vi "COMTRADE Open.vi"(5 "include information file? (F)":bool, 7 "include header file? (F)":bool, 8 "error in (no error)":errorcluster, 10 "open mode":T1(ring), 11 "configuration file path":path) -> (0 "error out":errorcluster, 3 "task out":T2 {"public inf content"."Event Information"."min sample number" max=9999999999; "public inf content"."Event Information"."max sample number" max=9999999999; "config info"."nrates" max=999; "config info"."status channel info"."Dn" min=1 max=999999; "config info"."analog channel info"."An" min=1 max=999999; "config info"."trigger timestamp" format="%<%H:%M:%S%6u\n%d/%m/%Y>T"; "config info"."initial timestamp" format="%<%H:%M:%S%6u\n%d/%m/%Y>T"; "config info"."##D" max=999999; "config info"."##A" max=999999; "config info"."TT" min=1 max=999999; "config info"."rev_year" min=1999.0 max=1999.0})   [LabVIEW 2013, in "NI_EP_COMTRADE.lvlib"]
doc: "Opens a .cfg and the corresponding .dat file for reading or writing. You also can use this VI to create a new file or replace an existing file. Set <B>include header file?</B> or <B>include information file?</B> to TRUE if you also want to create or open a .hdr or .inf file. Use the COMTRADE Close VI to close references to the files. IEEE Std C37.111-1999 specifies that a filename must not exceed eight characters. However, this VI accepts filenames that have more than eight characters, but returns a warning message."
uses:
  <vilib>/addons/Electrical Power/File IO/NI_EP_COMTRADE.lvlib
  <vilib>/addons/Electrical Power/File IO/COMTRADE/typedefs/ep_Task.ctl
  <vilib>/addons/Electrical Power/File IO/COMTRADE/typedefs/ep_Config Info.ctl
  <vilib>/addons/Electrical Power/File IO/COMTRADE/typedefs/ep_Analog Channel Info.ctl
  <vilib>/addons/Electrical Power/File IO/COMTRADE/typedefs/ep_Status Channel Info.ctl
  <vilib>/addons/Electrical Power/File IO/COMTRADE/typedefs/ep_File Format.ctl
  <vilib>/addons/Electrical Power/File IO/COMTRADE/typedefs/ep_Public Inf Content.ctl
  <vilib>/addons/Electrical Power/File IO/COMTRADE/typedefs/ep_Public Event Inf.ctl
  <vilib>/addons/Electrical Power/File IO/COMTRADE/typedefs/ep_Private Inf Content.ctl
  <vilib>/Platform/storage/lvStorage.llb/_openFunction.ctl
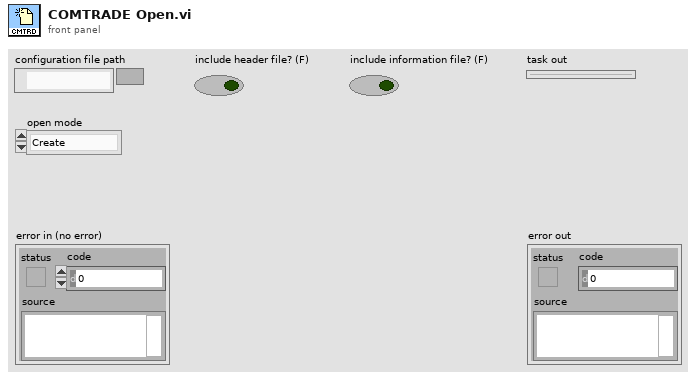
[diagram p1: front panel]
types:
  T1 = enum16{"Create", "Create or replace", "Open (read only)"}
  T2 = typedef "NI_EP_COMTRADE.lvlib/ep_Task.ctl" = cluster{"file refnums":refnum<file>[], "Data Object":refnum<k20>, "config info":T3, "public inf content":T7, "private inf content":T9, "internal buffers":cluster{"start index":u32, "config to public inf":enum16{"disabled", "enabled", "buffered"}, "static config info":string, "static file_des record inf":string, "static file_des channel inf":string, "public inf":string, "private inf":string}}
  T3 = typedef "NI_EP_COMTRADE.lvlib/ep_Config Info.ctl" = cluster{"station_name":string, "rec_dev_id":string, "rev_year":dbl, "TT":u32, "##A":u32, "##D":u32, "analog channel info":T4[], "status channel info":T5[], "lf":sgl, "nrates":u16, "samp info":cluster{"samp":sgl, "endsamp":u32}[], "initial timestamp":timestamp, "trigger timestamp":timestamp, "ft":T6, "timemult":sgl}
  T4 = typedef "NI_EP_COMTRADE.lvlib/ep_Analog Channel Info.ctl" = cluster{"An":u32, "ch_id":string, "ph":string, "ccbm":string, "uu":string, "a":sgl, "b":sgl, "skew":sgl, "min":i32, "max":i32, "primary":sgl, "secondary":sgl, "PS":enum16{"P", "S"}}
  T5 = typedef "NI_EP_COMTRADE.lvlib/ep_Status Channel Info.ctl" = cluster{"Dn":u32, "ch_id":string, "ph":string, "ccbm":string, "Y":bool}
  T6 = typedef "NI_EP_COMTRADE.lvlib/ep_File Format.ctl" = enum16{"ASCII", "Binary"}
  T7 = typedef "NI_EP_COMTRADE.lvlib/ep_Public Inf Content.ctl" = cluster{"Source":string, "Record Type":enum16{"Fault", "Unknown", "Misoperation", "Close", "Trip", "Reclose", "Power swing", "Simulation"}, "Phase ID":string, "Event Description":string, "Device ID":string, "Distance of Fault":dbl, "Distance Unit":enum16{"Miles", "Kilometers", "Percent of line", "Percent of setting", "Ohms"}, "Max_Current":dbl, "Min_Current":dbl, "Max_Voltage":dbl, "Min_Voltage":dbl, "EventNoteCount":u32, "Event Information":T8[]}
  T8 = typedef "NI_EP_COMTRADE.lvlib/ep_Public Event Inf.ctl" = cluster{"channel number":u32, "max value":dbl, "min value":dbl, "max sample number":u64, "min sample number":u64, "max sample text":string[], "min sample text":string[]}
  T9 = typedef "NI_EP_COMTRADE.lvlib/ep_Private Inf Content.ctl" = cluster{"Section Header":string, "Entry Names":string[], "Entry Values":string[]}[]
  T10 = enum16{"open", "replace", "create", "open or create", "replace or create", "replace or create with confirmation"}
  T11 = typedef "_openFunction.ctl" = enum16{"open", "open or create", "create or replace", "create", "open (read only)"}
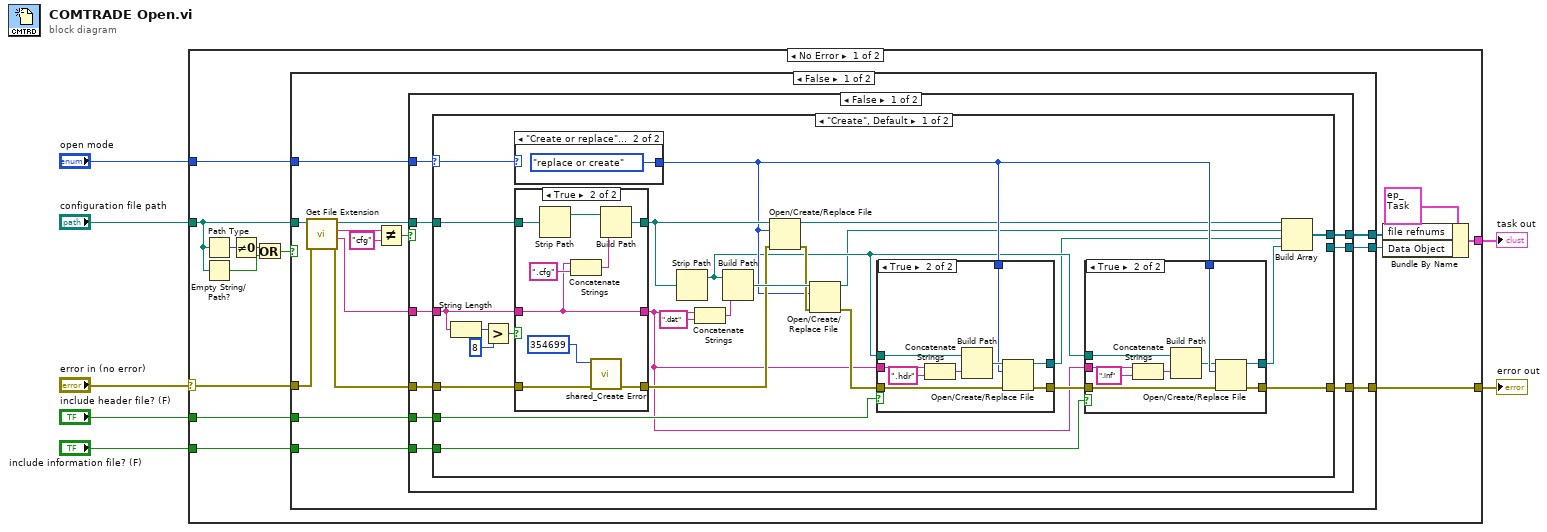
[diagram p0: block diagram]
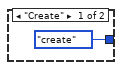
[diagram p2: hidden frame]
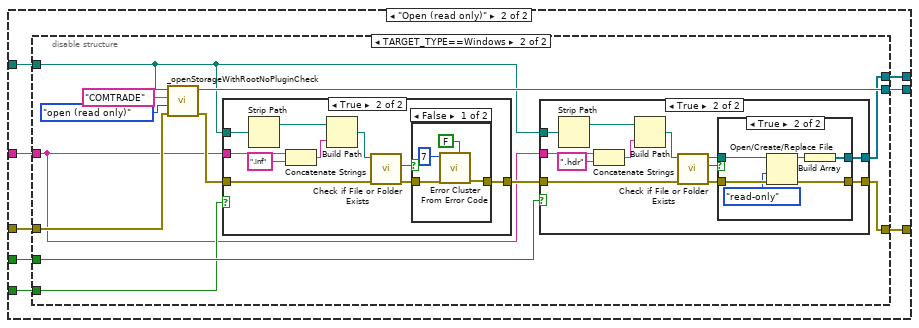
[diagram p6: hidden frame]
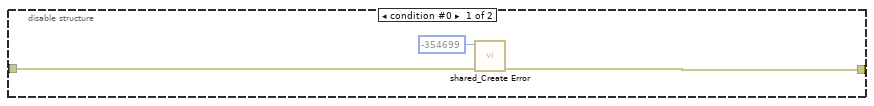
[diagram p7: hidden frame]
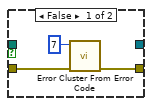
[diagram p11: hidden frame]
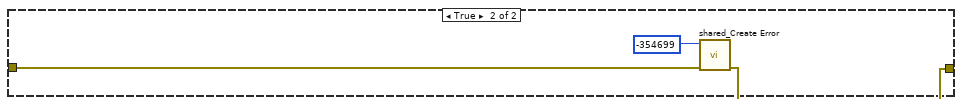
[diagram p12: hidden frame]
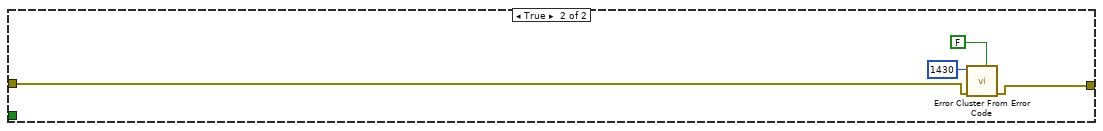
[diagram p13: hidden frame]
diagram:
  n1 = case shown="No Error" "error in (no error)" {
    selector: "error in (no error)" -> [w17 w173]
    tunnel: "open mode" -> [w16 _]
    tunnel: "configuration file path" -> [w9 _]
    tunnel: [w19 w173] -> w6
    tunnel: "include header file? (F)" -> [w21 _]
    tunnel: "include information file? (F)" -> [w20 _]
    tunnel: [w18 _] -> w2
    frame No Error {
      n2 = Path Type(1:w9) -> (0:w12:i16)
      n3 = Empty String/Path?(string/path=w9) -> (empty?=w10:bool)
      n4 = Not Equal To 0?(x=w12) -> (x != 0?=w11:bool)
      n5 = Or(x=w11, y=w10) -> (x .or. y?=w8:bool)
      n6 = case shown="False" w8 {
        tunnel: w21 -> [w35 _]
        tunnel: w20 -> [w34 _]
        tunnel: [w33 w170] -> w19
        tunnel: w17 -> [w29 w169]
        tunnel: w16 -> [w28 _]
        tunnel: [w25 _] -> w14
        tunnel: [w24 _] -> w13
        tunnel: w9 -> [w23 _]
        frame False {
          n7 = call <vilib>:"Get File Extension.vi"("error in (no error)"=w29, "file"=w23) -> ("error out"=w30:errorcluster, "filename without extension"=w31:string, "lowercase file extension"=w27:string, "dup file"=w32:path)  [unwired: 6 in]
          n8 = Not Equal?(x=w27, y="cfg") -> (x != y?=w22:bool)
          n9 = case shown="False" w22 {
            tunnel: w35 -> [w44 _]
            tunnel: w34 -> [w43 _]
            tunnel: [w42 w166] -> w33
            tunnel: w32 -> [w41 _]
            tunnel: w31 -> [w40 _]
            tunnel: w30 -> [w39 w167]
            tunnel: w28 -> [w38 _]
            tunnel: [w37 _] -> w25
            tunnel: [w36 _] -> w24
            frame False {
              n10 = case shown="\"Create\", Default" w38 {
                selector: w38 -> [w52 _]
                tunnel: w44 -> [w70 w106]
                tunnel: [w69 w110] -> w42
                tunnel: w40 -> [w66 w108]
                tunnel: w41 -> [w63 w109]
                tunnel: w39 -> [w56 w107]
                tunnel: [w45 w111] -> w37
                tunnel: w43 -> [w53 w105]
                tunnel: [_ w112] -> w36
                frame "Create", Default {
                  n11 = String Length(string=w66) -> (length=w68:i32)
                  n12 = Greater?(x=w68, y=8) -> (0:w67:bool)
                  n13 = case shown="\"Create or replace\", Default" w52 {
                    tunnel: [T10."create" ("operation (0:open)") T10."replace or create" ("operation (0:open)")] -> w51
                    frame "Create" {
                    }
                    frame "Create or replace", Default {
                    }
                  }
                  n14 = case shown="True" w67 {
                    tunnel: w66 -> [w75 w79]
                    tunnel: [w75 w79] -> w54
                    tunnel: w63 -> [w74 w83]
                    tunnel: [w74 w80] -> w62
                    tunnel: [w73 w76] -> w57
                    tunnel: w56 -> [w73 w77]
                    frame False {
                    }
                    frame True {
                      n15 = Strip Path(path=w83) -> (stripped path=w82:path)  [unwired: 1 out]
                      n16 = Concatenate Strings(w79, ".cfg" ("string")) -> (w81:string)
                      n17 = call <vilib>:"shared_Create Error.vi"("error in (no error)"=w77, "error code (0)"=354699 ("code")) -> ("error out"=w76:errorcluster)  [unwired: 9 in]
                      n18 = Build Path(base path=w82, name or relative path=w81) -> (appended path=w80:path)
                    }
                  }
                  n19 = Strip Path(path=w62) -> (stripped path=w50:path)  [unwired: 1 out]
                  n20 = Concatenate Strings(w54, ".dat" ("string")) -> (w61:string)
                  n21 = Build Path(base path=w50, name or relative path=w61) -> (appended path=w60:path)
                  n22 = Open/Create/Replace File(file path (use dialog)=w62, error in=w57, operation (0:open)=w51) -> (refnum out=w49:refnum<file>, error out=w59:errorcluster)  [unwired: 3 in, 1 out]
                  n23 = Open/Create/Replace File(file path (use dialog)=w60, error in=w59, operation (0:open)=w51) -> (refnum out=w48:refnum<file>, error out=w58:errorcluster)  [unwired: 3 in, 1 out]
                  n24 = case shown="True" w70 {
                    tunnel: w54 -> [_ w100]
                    tunnel: w51 -> [_ w103]
                    tunnel: w58 -> [w95 w99]
                    tunnel: [w95 w98] -> w55
                    tunnel: w50 -> [_ w97]
                    tunnel: [_ w96] -> w47
                    frame False {
                    }
                    frame True {
                      n25 = Concatenate Strings(w100, ".hdr" ("string")) -> (w101:string)
                      n26 = Build Path(base path=w97, name or relative path=w101) -> (appended path=w104:path)
                      n27 = Open/Create/Replace File(file path (use dialog)=w104, error in=w99, operation (0:open)=w103) -> (refnum out=w96:refnum<file>, error out=w98:errorcluster)  [unwired: 3 in, 1 out]
                    }
                  }
                  n28 = case shown="True" w53 {
                    tunnel: w54 -> [_ w90]
                    tunnel: w51 -> [_ w94]
                    tunnel: [w85 w93] -> w69
                    tunnel: w55 -> [w85 w89]
                    tunnel: w50 -> [_ w87]
                    tunnel: [_ w86] -> w46
                    frame False {
                    }
                    frame True {
                      n29 = Concatenate Strings(w90, ".inf" ("string")) -> (w92:string)
                      n30 = Build Path(base path=w87, name or relative path=w92) -> (appended path=w91:path)
                      n31 = Open/Create/Replace File(file path (use dialog)=w91, error in=w89, operation (0:open)=w94) -> (refnum out=w86:refnum<file>, error out=w93:errorcluster)  [unwired: 3 in, 1 out]
                    }
                  }
                  n32 = Build Array(w49, w48, w47, w46) -> (w45:refnum<file>[])
                }
                frame "Open (read only)" {
                  n33 = disable-structure shown="TARGET_TYPE==Windows" {
                    disable-tunnel: [_ w123] -> w112
                    disable-tunnel: [_ w122] -> w111
                    disable-tunnel: [w114 w121] -> w110
                    disable-tunnel: w109 -> [_ w120]
                    disable-tunnel: w108 -> [_ w116]
                    disable-tunnel: w107 -> [w115 w119]
                    disable-tunnel: w106 -> [_ w118]
                    disable-tunnel: w105 -> [_ w117]
                    frame condition #0 {
                      n34 = call <vilib>:"shared_Create Error.vi"("error in (no error)"=w115, "error code (0)"=-354699) -> ("error out"=w114:errorcluster)  [unwired: 9 in]
                    }
                    frame condition #1 (active) {
                      n35 = call <vilib>:"_openStorageWithRootNoPluginCheck.vi"("error in (no error)"=w119, "Overwrite Options"=_openFunction."open (read only)", "Storage Format"="COMTRADE", "Storage Location"=w120) -> ("error out"=w126:errorcluster, "Data Object"=w123:refnum<k20>)  [unwired: 6 in]
                      n36 = case shown="True" w117 {
                        tunnel: w116 -> [_ w137]
                        tunnel: [w128 w131] -> w127
                        tunnel: w126 -> [w128 w134]
                        tunnel: w120 -> [_ w130]
                        frame False {
                        }
                        frame True {
                          n37 = Strip Path(path=w130) -> (stripped path=w129:path)  [unwired: 1 out]
                          n38 = Concatenate Strings(w137, ".inf" ("string")) -> (w138:string)
                          n39 = Build Path(base path=w129, name or relative path=w138) -> (appended path=w135:path)
                          n40 = call <vilib>:"Check if File or Folder Exists.vi"("error in (no error)"=w134, "path"=w135) -> ("error out"=w132:errorcluster, "file or folder exists?"=w133:bool)  [unwired: 7 in, 1 out]
                          n41 = case shown="False" w133 {
                            tunnel: w132 -> [w142 w143]
                            tunnel: [w141 w143] -> w131
                            frame False {
                              n42 = call <vilib>:"Error Cluster From Error Code.vi"("is warning? (False)"=FALSE, "error in (no error)"=w142, "error code (0)"=7) -> ("error out"=w141:errorcluster)  [unwired: 6 in]
                            }
                            frame True {
                            }
                          }
                        }
                      }
                      n43 = case shown="True" w118 {
                        tunnel: w120 -> [_ w153]
                        tunnel: w116 -> [_ w154]
                        tunnel: w127 -> [w144 w148]
                        tunnel: [w144 w147] -> w121
                        tunnel: [_ w145] -> w122
                        frame False {
                        }
                        frame True {
                          n44 = Strip Path(path=w153) -> (stripped path=w152:path)  [unwired: 1 out]
                          n45 = Concatenate Strings(w154, ".hdr" ("string")) -> (w156:string)
                          n46 = Build Path(base path=w152, name or relative path=w156) -> (appended path=w149:path)
                          n47 = call <vilib>:"Check if File or Folder Exists.vi"("error in (no error)"=w148, "path"=w149) -> ("error out"=w150:errorcluster, "file or folder exists?"=w151:bool, "dup path"=w146:path)  [unwired: 7 in]
                          n48 = case shown="True" w151 {
                            tunnel: w150 -> [w158 w164]
                            tunnel: [w159 w163] -> w147
                            tunnel: w146 -> [_ w162]
                            tunnel: [_ w161] -> w145
                            frame False {
                              n49 = call <vilib>:"Error Cluster From Error Code.vi"("error in (no error)"=w158, "error code (0)"=7) -> ("error out"=w159:errorcluster)  [unwired: 7 in]
                            }
                            frame True {
                              n50 = Open/Create/Replace File(file path (use dialog)=w162, error in=w164, access (0:read/write)=enum16{"read/write", "read-only", "write-only"}."read-only") -> (refnum out=w165:refnum<file>, error out=w163:errorcluster)  [unwired: 3 in, 1 out]
                              n51 = Build Array(w165) -> (w161:refnum<file>[])
                            }
                          }
                        }
                      }
                    }
                  }
                }
              }
            }
            frame True {
              n52 = call <vilib>:"shared_Create Error.vi"("error in (no error)"=w167, "error code (0)"=-354699 ("code")) -> ("error out"=w166:errorcluster)  [unwired: 9 in]
            }
          }
        }
        frame True {
          n53 = call <vilib>:"Error Cluster From Error Code.vi"("is warning? (False)"=FALSE, "error in (no error)"=w169, "error code (0)"=1430) -> ("error out"=w170:errorcluster)  [unwired: 6 in]
        }
      }
      n54 = Bundle By Name(cluster=T2 {"file refnums"=[], "Data Object"=refnum, "config info"={"station_name"="", "rec_dev_id"="", "rev_year"=0.0, "TT"=0, "##A"=0, "##D"=0, "analog channel info"=[], "status channel info"=[], "lf"=0.0, "nrates"=0, "samp info"=[], "initial timestamp"=timestamp(0 s since 1904-01-01), "trigger timestamp"=timestamp(0 s since 1904-01-01), "ft"=enum."ASCII", "timemult"=0.0}, "public inf content"={"Source"="", "Record Type"=enum."Fault", "Phase ID"="", "Event Description"="", "Device ID"="", "Distance of Fault"=0.0, "Distance Unit"=enum."Miles", "Max_Current"=0.0, "Min_Current"=0.0, "Max_Voltage"=0.0, "Min_Voltage"=0.0, "EventNoteCount"=0, "Event Information"=[]}, "private inf content"=[], "internal buffers"={"start index"=1, "config to public inf"=enum."disabled", "static config info"="", "static file_des record inf"="", "static file_des channel inf"="", "public inf"="", "private inf"=""}} ("task out"), "file refnums"=w14, "Data Object"=w13) -> (w18:T2)
    }
    frame Error {
    }
  }
  "error out" <- w6
  "task out" <- w2
